vi "ESP Send.vi"(4 "error in":errorcluster, 5 "Command String":string, 7 "Address / Port":i16=1 min=1 max=31 step=1) -> (0 "error out":errorcluster, 3 "Address / Port dup":i16=1 min=1 max=31 step=1)   [LabVIEW 2014]
panel:
  out "status":bool[](array[boolean])
  out "byte count":i32
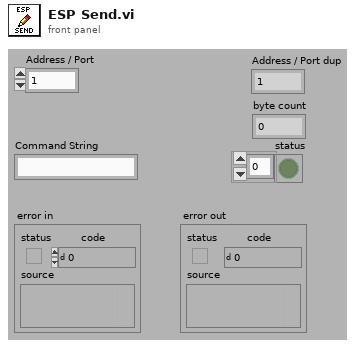
[diagram p1: front panel]
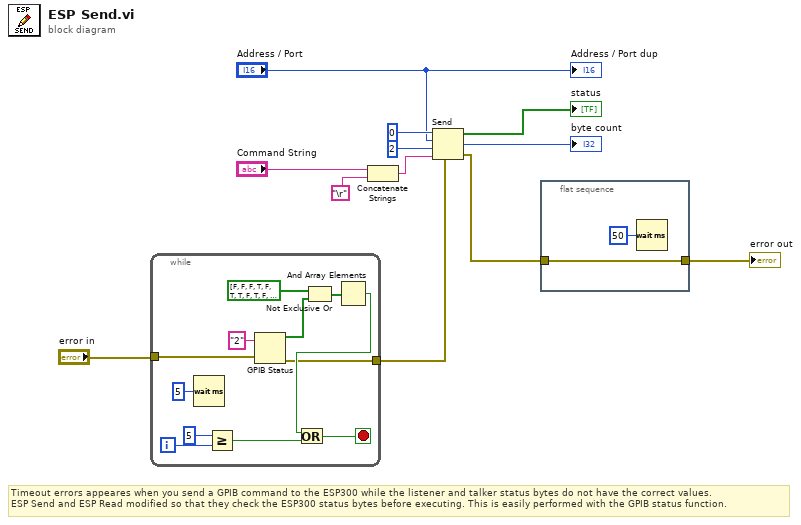
[diagram p0: block diagram]
diagram:
  # "Timeout errors appeares when you send a GPIB command to the ESP300 while the listener and talker status bytes do not have the correct values.\nESP Send and ESP Read modified so that they check the ESP300 status bytes before executing. This is easily performed with the GPIB status function."
  n1 = while {
    tunnel: "error in" -> [w23]
    tunnel: [w13] -> w3
    i -> [w22]
    stop <- w19 stop-if-true
    n2 = Wait (ms)(milliseconds to wait=u32 5) -> ()  [unwired: 1 out]
    n3 = Greater Or Equal?(x=5, y=w22) -> (x >= y?=w20:bool)
    n4 = GPIB Status(0:"2" ("address string"), 1:w23) -> (2:w17:bool[], 5:w13:errorcluster)  [unwired: 2 out]
    n5 = Not Exclusive Or(1:w17, 2:bool[] [FALSE, FALSE, FALSE, TRUE, FALSE, TRUE, TRUE, FALSE, TRUE, FALSE, FALSE, FALSE, FALSE, FALSE, FALSE, FALSE] ("status 2")) -> (0:w16:bool[])
    n6 = And Array Elements(Boolean array=w16) -> (logical AND=w15:bool)
    n7 = Or(x=w15, y=w20) -> (x .or. y?=w19:bool)
  }
  n8 = Concatenate Strings("Command String", "\r") -> (w9:string)
  n9 = Send(0:0 ("bus"), 2:"Address / Port", 3:i16 2 ("mode"), 4:w3, 5:w9) -> (6:→"status":bool[], 7:→"byte count":i32, 8:w2:errorcluster)
  n10 = flat-sequence {
    tunnel: w2 -> [w25]
    tunnel: [w25] -> w1
    frame #0 {
      n11 = Wait (ms)(milliseconds to wait=u32 50) -> ()  [unwired: 1 out]
    }
  }
  "error out" <- w1
  "Address / Port dup" <- "Address / Port"
